vi "Main UI.vi"() -> ()   [LabVIEW 2021]
uses:
  subVIs/TypeDefs/UIControlReferences.ctl
  subVIs/TypeDefs/Tester Object.ctl
  <vilib>/NI/Modbus Library/API/Master/Modbus Master.lvclass
  <vilib>/Utility/error.llb/DialogType.ctl
panel:
  in  "Connect":bool
  in  "Stop Process":bool
  out "Equipment Status":bool caption="Equipment Connection"
  out "Positioning":dbl
  out "Motor Speed":dbl
  out "Temperature":dbl
  in  "ctrlCalibrate":bool
  out "Calibration":bool caption="Calibrated"
  in  "Sensibility Adjust":dbl caption="Sensibility"
  in  "ctrlSettingsButton":bool caption="Settings Button"
  in  "ctrlDirectionRotation":bool caption="Direction of Rotation"
  in  "ctrlMotorControlMode":bool caption="Motor Control Mode"
  in  "ctrlMotorControl":u16 caption="Motor Control (rpm)"
  in  "ctrlElevatorPosition":u16 caption="Elevator Position"
  in  "setShearRampStep":bool caption="Shear Ramp Step"
  in  "setOscillatory":bool caption="Oscillatory"
  in  "setShearRamp":bool caption="Shear Ramp"
  in  "setRTConstant":bool caption="Rotation or Torque Constant"
  in  "setElevatorPosition":bool caption="Set Elevator Position"
  in  "seqPauseButton":bool
  in  "Save Button":bool
  in  "stopJobSequence":bool
  in  "startJobSequence":bool
  in  "Data Analysis":bool
  in  "Job Sequence Tree":string(tree) caption="Job Sequence"
  out "XY Graph":cluster{dbl[], dbl[]}[](graph)
  out "Sensors":string[][](table)=[["Speed (rpm)", "125,6"], ["Torque (Nm)", "-0,301"], ["Height (mm)", "36"], ["Samples/s", "10,0"], ["Duration (s)", "250,4"]]
  out "Status String 3":string
  out "Status String 1":string
  out "Status String 2":string
  # "Equipment"
  # "Job Selection"
  # "Data Analysis"
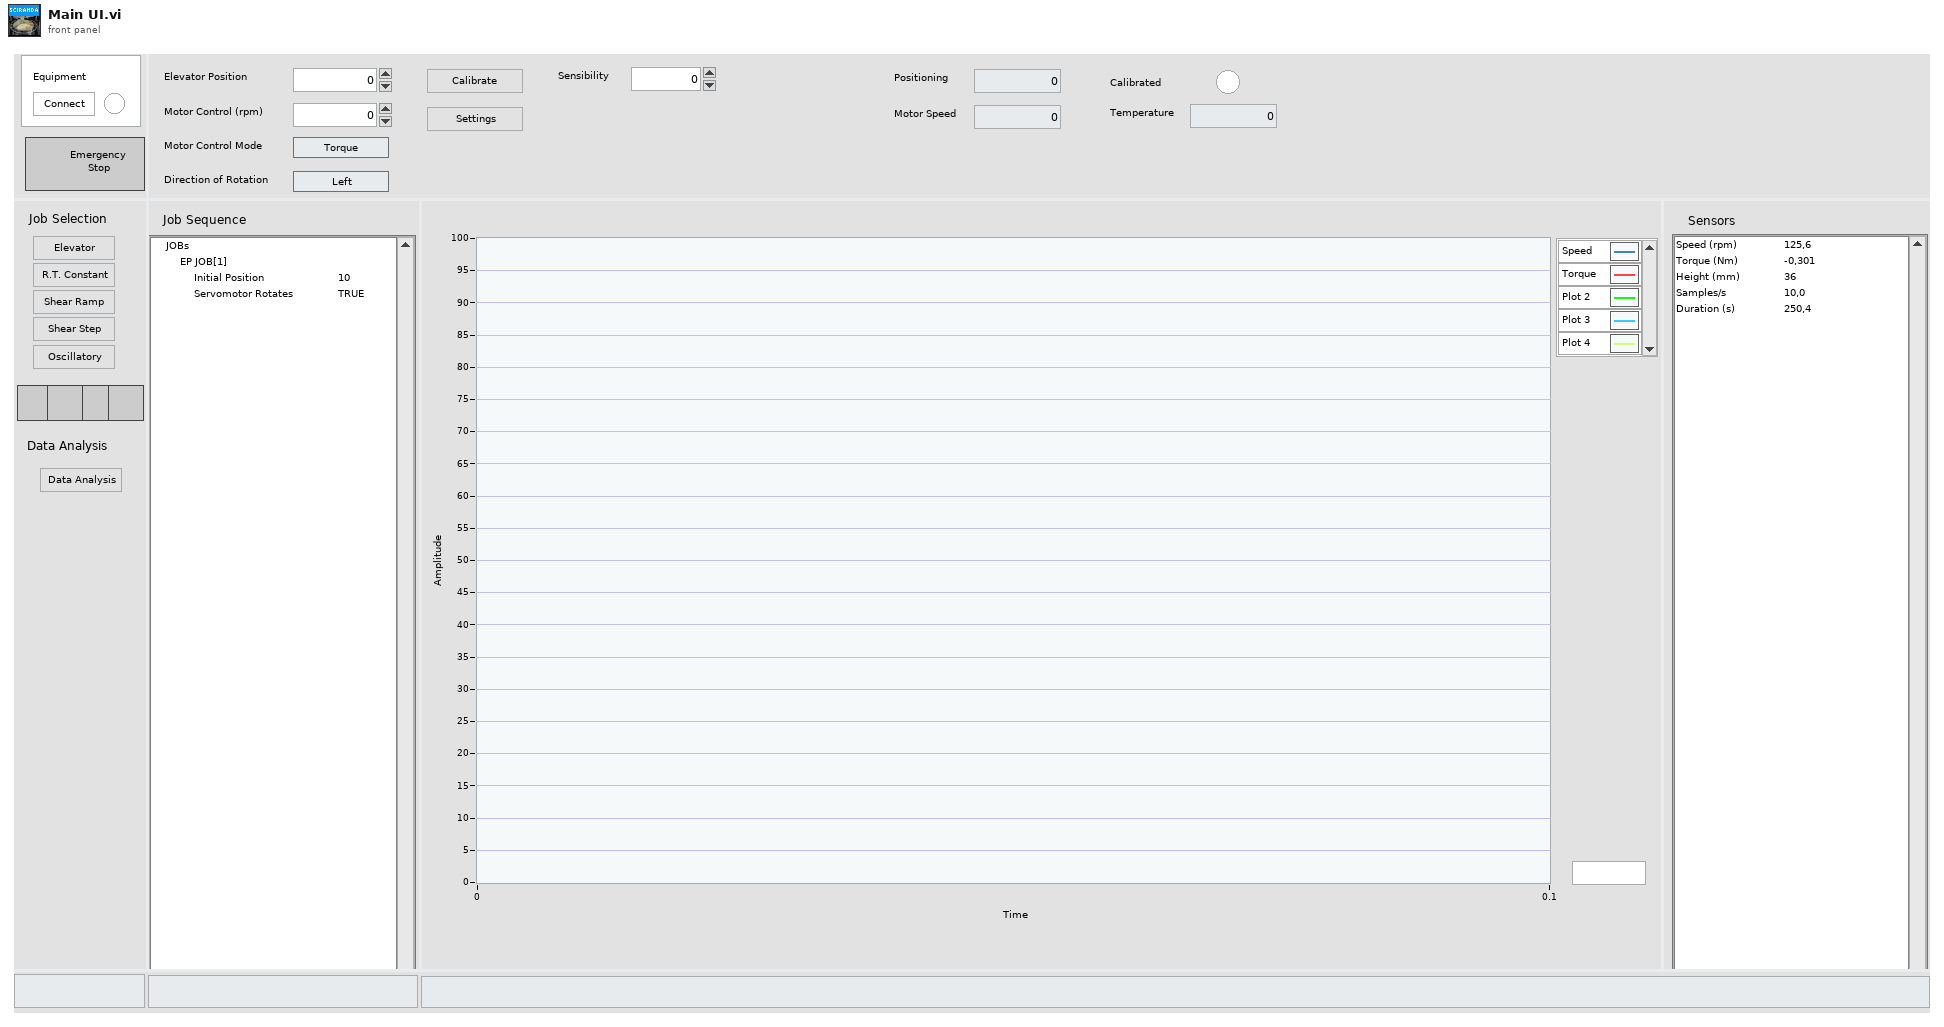
[diagram p1: front panel]
types:
  T1 = typedef "Tester Object.ctl" = cluster{"Program Properties":cluster{"Application Path":path}, "Control Refnum":T2, "Devices":cluster{"Modbus":cluster{"Modbus master instance":refnum<class "Modbus Master.lvclass">, "Modbus Address":cluster{"Session":string, cluster{"Key":string, "value":u32}[]}[]}, "TCP/IP":cluster{"connection ID":refnum<k5>, "Address":string}}}
  T2 = typedef "UIControlReferences.ctl" = cluster{"Tree Refnum ":refnum<vi>, "Graph1 Refnum":refnum<vi>, "Graph2 Refnum":refnum<vi>, "Temperature Refnum":refnum<vi>, "Sensor Str Refnum":refnum<vi>, "Motor Speed Refnum":refnum<vi>, "Equipment Connected Refnum":refnum<vi>, "Calibrated Refnum":refnum<vi>, "Positioning Refnum":refnum<vi>, "Servo On Refnum":refnum<vi>, "seqPauseButton":refnum<vi>, "seqStartButton":refnum<vi>, "seqStopButton":refnum<vi>}
  T3 = cluster{"Session":string, cluster{"Key":string, "value":u32}[]}[]
  T4 = typedef "DialogType.ctl" = u16
  T5 = cluster{"Modbus":cluster{"Modbus master instance":refnum<class "Modbus Master.lvclass">, "Modbus Address":cluster{"Session":string, cluster{"Key":string, "value":u32}[]}[]}, "TCP/IP":cluster{"connection ID":refnum<k5>, "Address":string}}
  T6 = typedef "ElevatorPositionConfiguration.ctl" = cluster{"ElevatorStartPosition":dbl, "ServomotorRotates":bool, "ElevatorPositionConfirmed?":bool}
  T7 = typedef "RotateOrTorqueConstantConfiguration.ctl" = cluster{"Constant Value":dbl, "Rotation or Torque":string, "Duration":dbl, "Confirmed?":bool}
  T8 = typedef "ShearRampConfiguration.ctl" = cluster{"Shear Ramp":string, "Rotation or Torque":string, "Initial Value":dbl, "Final Value":dbl, "Duration":dbl, "Number of Points":i32, "Confirmed?":bool, "Shear Ramp Array":dbl[][]}
  T9 = typedef "ShearRampStepConfiguration.ctl" = cluster{"Rotation or Torque":string, "Initial Value":dbl, "Final Value":dbl, "Step Duration":dbl, "Number of Steps":i32, "Shear Ramp Step Array":dbl[][], "Confirmed?":bool, "Shear Step Generation":enum16{"StepDurationConstant", "Table"}}
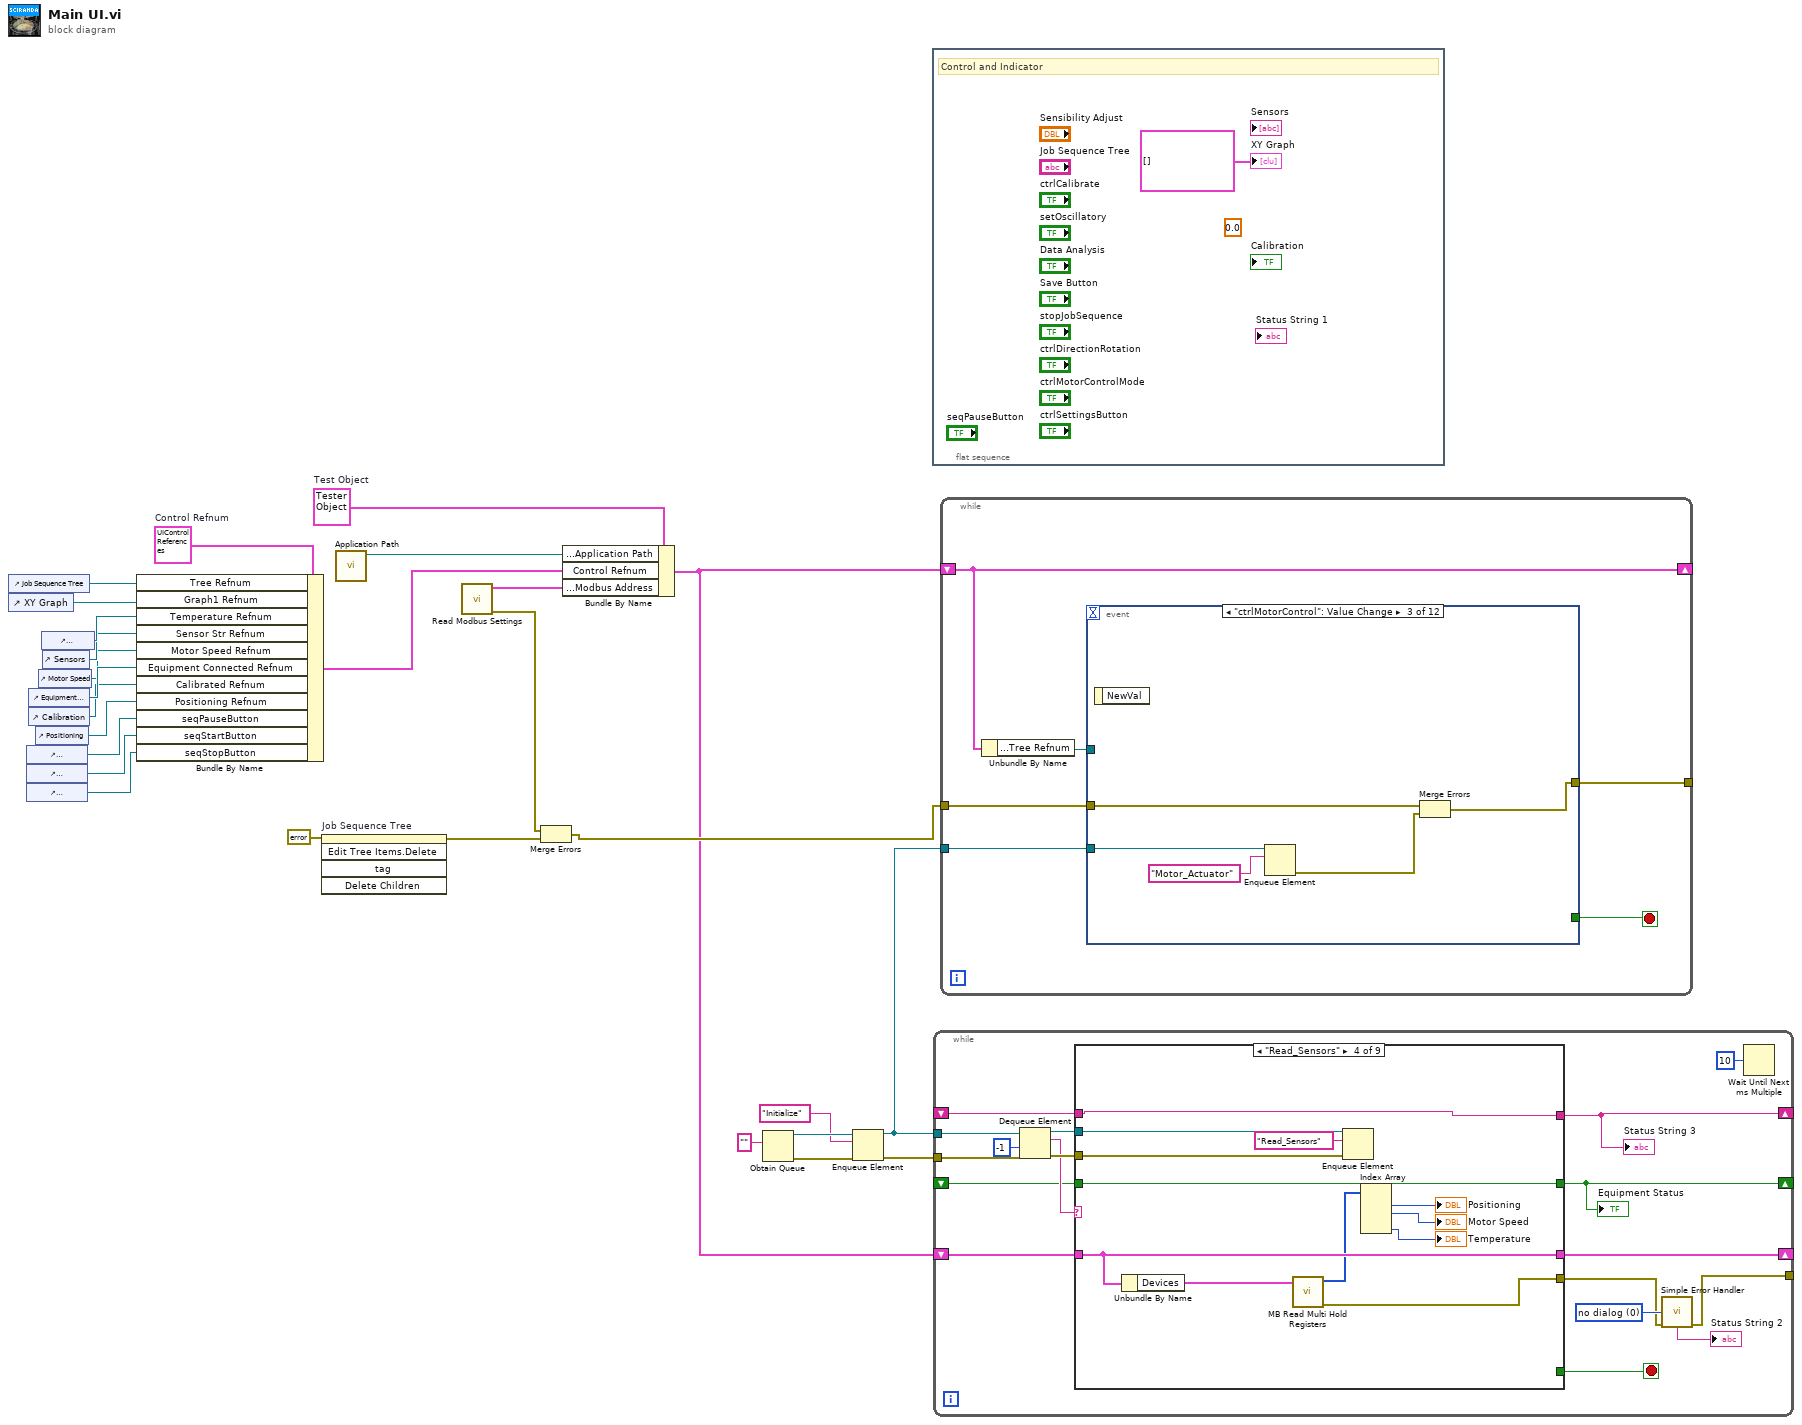
[diagram p0: block diagram]
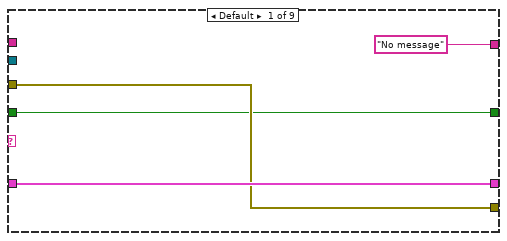
[diagram p2: hidden frame]
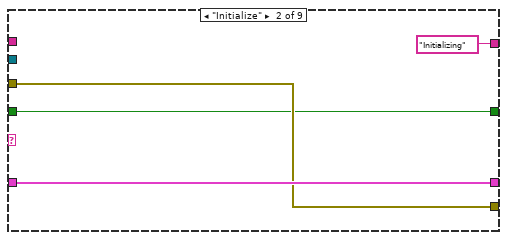
[diagram p3: hidden frame]
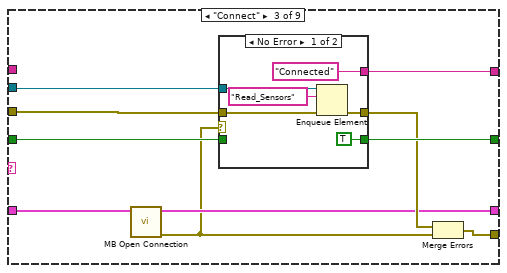
[diagram p4: hidden frame]
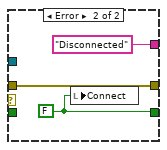
[diagram p5: hidden frame]
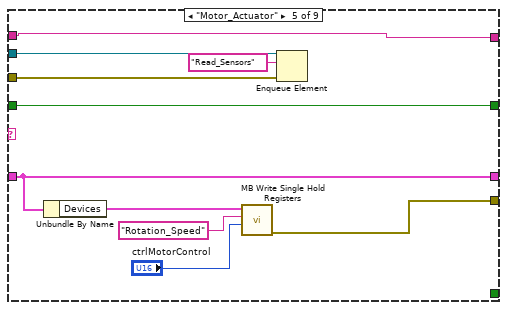
[diagram p6: hidden frame]
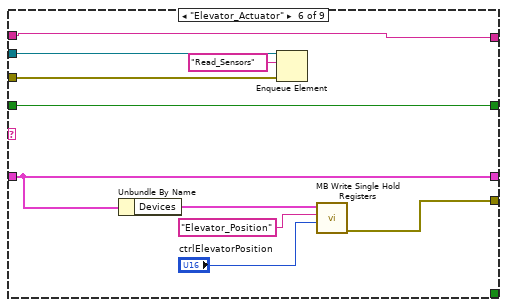
[diagram p7: hidden frame]
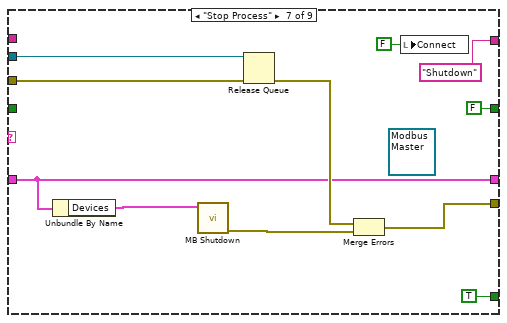
[diagram p8: hidden frame]
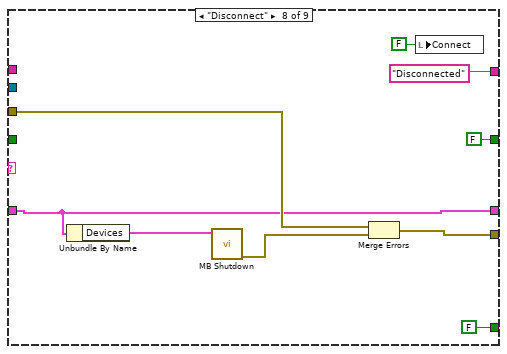
[diagram p9: hidden frame]
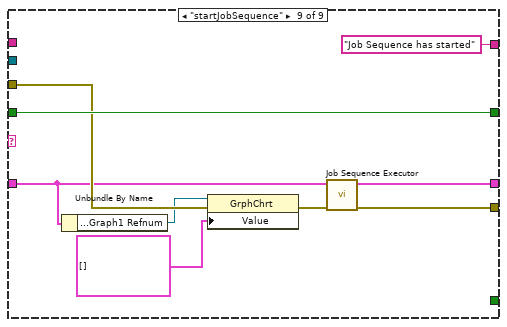
[diagram p10: hidden frame]
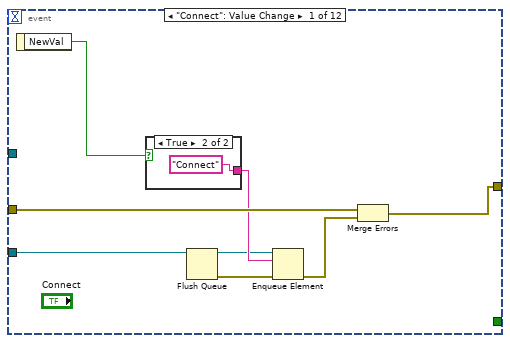
[diagram p11: hidden frame]
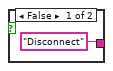
[diagram p12: hidden frame]
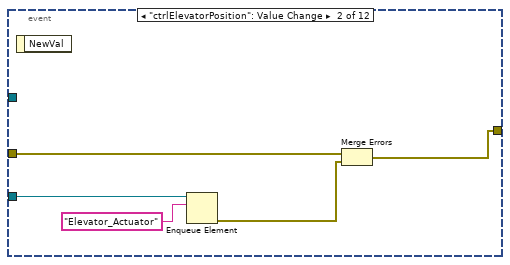
[diagram p13: hidden frame]
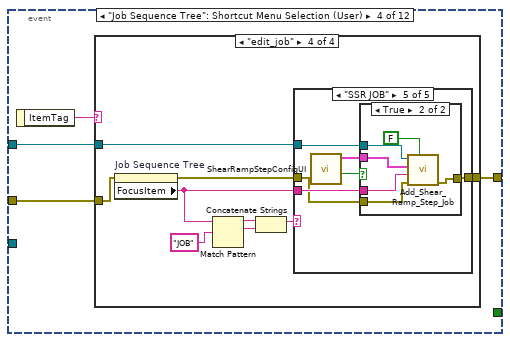
[diagram p14: hidden frame]
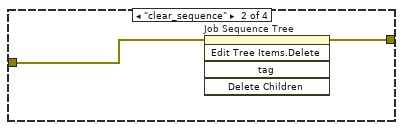
[diagram p16: hidden frame]
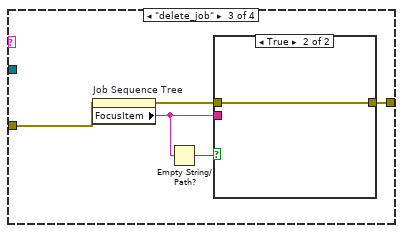
[diagram p17: hidden frame]
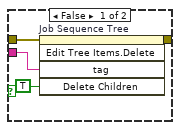
[diagram p18: hidden frame]
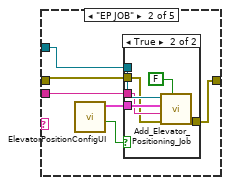
[diagram p20: hidden frame]
diagram:
  w10 = T1 {"Program Properties"={"Application Path"=path ""}, "Control Refnum"={"Tree Refnum "=refnum, "Graph1 Refnum"=refnum, "Graph2 Refnum"=refnum, "Temperature Refnum"=refnum, "Sensor Str Refnum"=refnum, "Motor Speed Refnum"=refnum, "Equipment Connected Refnum"=refnum, "Calibrated Refnum"=refnum, "Positioning Refnum"=refnum, "Servo On Refnum"=refnum, "seqPauseButton"=refnum, "seqStartButton"=refnum, "seqStopButton"=refnum}, "Devices"={"Modbus"={"Modbus master instance"=refnum, "Modbus Address"=[]}, "TCP/IP"={"connection ID"=refnum, "Address"=""}}}  # Test Object
  w20 = T2 {"Tree Refnum "=refnum, "Graph1 Refnum"=refnum, "Graph2 Refnum"=refnum, "Temperature Refnum"=refnum, "Sensor Str Refnum"=refnum, "Motor Speed Refnum"=refnum, "Equipment Connected Refnum"=refnum, "Calibrated Refnum"=refnum, "Positioning Refnum"=refnum, "Servo On Refnum"=refnum, "seqPauseButton"=refnum, "seqStartButton"=refnum, "seqStopButton"=refnum}  # Control Refnum
  n1 = control-ref of="Job Sequence Tree"() -> (w19:refnum<vi>)
  n2 = control-ref of="XY Graph"() -> (w14:refnum<vi>)
  n3 = control-ref of="seqPauseButton"() -> (w3:refnum<vi>)
  n4 = control-ref of="startJobSequence"() -> (w2:refnum<vi>)
  n5 = control-ref of="stopJobSequence"() -> (w1:refnum<vi>)
  n6 = control-ref of="Equipment Status"() -> (w16:refnum<vi>)
  n7 = control-ref of="Calibration"() -> (w15:refnum<vi>)
  n8 = control-ref of="Positioning"() -> (w5:refnum<vi>)
  n9 = control-ref of="Motor Speed"() -> (w4:refnum<vi>)
  n10 = control-ref of="Temperature"() -> (w18:refnum<vi>)
  n11 = control-ref of="Sensors"() -> (w17:refnum<vi>)
  n12 = Bundle By Name(cluster=w20, "Tree Refnum"=w19, "Graph1 Refnum"=w14, "Temperature Refnum"=w18, "Sensor Str Refnum"=w17, "Motor Speed Refnum"=w4, "Equipment Connected Refnum"=w16, "Calibrated Refnum"=w15, "Positioning Refnum"=w5, "seqPauseButton"=w3, "seqStartButton"=w2, "seqStopButton"=w1) -> (w9:T2)
  n13 = invoke on="Job Sequence Tree" class="Tree (strict)" method="Edit Tree Items.Delete"(error in=errorcluster {"status"=FALSE, "code"=0, "source"=""} ("error out")) -> (error out=w12:errorcluster)  [unwired: 4 in, 4 out]
  n14 = call "Application Path.vi"() -> ("appended path"=w7:path)  [unwired: 11 in]
  n15 = call "Read Modbus Settings.vi"() -> ("error out"=w11:errorcluster, "Ini File"=w6:T3)  [unwired: 10 in]
  n16 = Merge Errors(w11, w12) -> (w27:errorcluster)
  n17 = Bundle By Name(cluster=w10, "Program Properties.Application Path"=w7, "Control Refnum"=w9, "Devices.Modbus.Modbus Address"=w6) -> (w8:T1)
  n18 = Obtain Queue(element data type="" ("element")) -> (queue out=w26:refnum<queue>, error out=w24:errorcluster)  [unwired: 4 in, 1 out]
  n19 = Enqueue Element(queue=w26, element="Initialize", error in (no error)=w24) -> (queue out=w21:refnum<queue>, error out=w22:errorcluster)  [unwired: 1 in, 1 out]
  n20 = flat-sequence {
    frame #0 {
      (unwired) 0.0 ("Temperature")
      # "Control and Indicator"
      "XY Graph" <- cluster{dbl[], dbl[]}[] [] ("Multiplot XY Array")
    }
  }
  n21 = while {
    shift-right: [w45] -> _
    shift-left: w8 -> [w46]
    tunnel: w21 -> [w44]
    tunnel: w22 -> [w43]
    shift-right: [w38] -> _
    shift-left: _ -> [w37]
    tunnel: [w33] -> _
    shift-right: [w32] -> _
    shift-left: _ -> [w31]
    stop <- w39 stop-if-true
    w35 = T4 0 items=["no dialog", "OK message", "continue or stop message", "OK message + warnings", "continue/stop + warnings"] ("type of dialog (OK msg:1)")
    n22 = Dequeue Element(queue=w44, timeout in ms (-1)=-1, error in (no error)=w43) -> (queue out=w41:refnum<queue>, element=w40:string, error out=w42:errorcluster)  [unwired: 1 out]
    n23 = case shown="\"Read_Sensors\"" w40 {
      tunnel: w46 -> [w50 w54 w57 w80 w89 w98 w106 w117 w127]
      tunnel: [w48 w52 w63 w74 w95 w97 w115 w125 w132] -> w34
      tunnel: [w50 w54 w56 w80 w89 w98 w106 w117 w128] -> w45
      tunnel: w42 -> [w48 w52 w59 w82 w91 w102 w110 w120 w131]
      tunnel: w41 -> [_ _ w60 w83 w92 w103 w108 _ _]
      tunnel: ["No message" "Initializing" w64 w85 w94 w105 "Shutdown" "Disconnected" "Job Sequence has started"] -> w32
      tunnel: [_ _ _ _ _ _ TRUE FALSE _] -> w39
      tunnel: [w47 w51 w62 w84 w93 w104 FALSE FALSE w134] -> w38
      tunnel: w37 -> [w47 w51 w61 w84 w93 w104 _ _ w134]
      tunnel: w31 -> [_ _ _ w85 w94 w105 _ _ _]
      frame Default {
      }
      frame "Initialize" {
      }
      frame "Connect" {
        n24 = call "MB Open Connection.vi"("Test Object in"=w57) -> ("error out"=w55:errorcluster, "Test Object out"=w56:T1)  [unwired: 9 in]
        n25 = case shown="No Error" w55 {
          tunnel: ["Connected" "Disconnected"] -> w64
          tunnel: [TRUE w71] -> w62
          tunnel: w61 -> [_ _]
          tunnel: w60 -> [w68 _]
          tunnel: w59 -> [w67 w72]
          tunnel: [w65 w72] -> w58
          frame No Error {
            n26 = Enqueue Element(queue=w68, element="Read_Sensors", error in (no error)=w67) -> (error out=w65:errorcluster)  [unwired: 1 in, 2 out]
          }
          frame Error {
            w71 = FALSE
            n27 = local write "Connect"(w71) -> ()
          }
        }
        n28 = Merge Errors(w58, w55) -> (w63:errorcluster)
      }
      frame "Read_Sensors" {
        n29 = Unbundle By Name(w80) -> ("Devices"=w79:T5)
        n30 = call "MB Read Multi Hold Registers.vi"("Devices"=w79) -> ("error out"=w74:errorcluster, "Register Values"=w78:u16[])  [unwired: 9 in]
        n31 = Enqueue Element(queue=w83, element="Read_Sensors", error in (no error)=w82) -> ()  [unwired: 1 in, 3 out]
        n32 = Index Array(array=w78) -> (element #1=→"Positioning":u16, element #2=→"Motor Speed":u16, element #4=→"Temperature":u16)  [unwired: 4 in, 1 out]
      }
      frame "Motor_Actuator" {
        n33 = Unbundle By Name(w89) -> ("Devices"=w88:T5)
        n34 = call "MB Write Single Hold Registers.vi"("Write Hold Register"="ctrlMotorControl", "Control Variable"="Rotation_Speed", "Devices"=w88) -> ("error out"=w95:errorcluster)  [unwired: 7 in, 1 out]
        n35 = Enqueue Element(queue=w92, element="Read_Sensors", error in (no error)=w91) -> ()  [unwired: 1 in, 3 out]
      }
      frame "Elevator_Actuator" {
        n36 = Unbundle By Name(w98) -> ("Devices"=w100:T5)
        n37 = Enqueue Element(queue=w103, element="Read_Sensors", error in (no error)=w102) -> ()  [unwired: 1 in, 3 out]
        n38 = call "MB Write Single Hold Registers.vi"("Write Hold Register"="ctrlElevatorPosition", "Control Variable"="Elevator_Position", "Devices"=w100) -> ("error out"=w97:errorcluster)  [unwired: 7 in, 1 out]
      }
      frame "Stop Process" {
        (unwired) refnum<class "Modbus Master.lvclass"> refnum ("TCP master instance")
        n39 = Unbundle By Name(w106) -> ("Devices"=w107:T5)
        n40 = call "MB Shutdown.vi"("Devices"=w107) -> ("error out"=w116:errorcluster)  [unwired: 10 in]
        n41 = Release Queue(queue=w108, error in (no error)=w110) -> (error out=w109:errorcluster)  [unwired: 1 in, 2 out]
        n42 = Merge Errors(w109, w116) -> (w115:errorcluster)
        n43 = local write "Connect"(FALSE ("Connect")) -> ()
      }
      frame "Disconnect" {
        n44 = Unbundle By Name(w117) -> ("Devices"=w119:T5)
        n45 = call "MB Shutdown.vi"("Devices"=w119) -> ("error out"=w118:errorcluster)  [unwired: 10 in]
        n46 = Merge Errors(w120, w118) -> (w125:errorcluster)
        n47 = local write "Connect"(FALSE ("Connect")) -> ()
      }
      frame "startJobSequence" {
        n48 = Unbundle By Name(w127) -> ("Control Refnum.Graph1 Refnum"=w126:refnum<vi>)
        n49 = property class="GrphChrt"(reference=w126, error in=w131, "Value"=cluster{dbl[], dbl[]}[] [] ("Multiplot XY Array")) -> (error out=w130:errorcluster)  [unwired: 1 out]
        n50 = call "Job Sequence Executor.vi"("error out"=w130, "Test Object"=w127) -> ("error out 2"=w132:errorcluster, "Test Object out"=w128:T1)  [unwired: 8 in]
      }
    }
    "Equipment Status" <- w38
    "Status String 3" <- w32
    n51 = call <vilib>:"Simple Error Handler.vi"("type of dialog (OK msg:1)"=w35, "error in (no error)"=w34) -> ("error out"=w33:errorcluster, "message"=→"Status String 2":string)  [unwired: 3 in, 3 out]
    n52 = Wait Until Next ms Multiple(millisecond multiple=u32 10) -> ()  [unwired: 1 out]
  }
  n53 = while {
    tunnel: [w139] -> _
    tunnel: w27 -> [w138]
    tunnel: w21 -> [w137]
    shift-right: [w135] -> _
    shift-left: w8 -> [w135]
    stop <- w140 stop-if-true
    n54 = Unbundle By Name(w135) -> ("Control Refnum.Tree Refnum"=w136:refnum<vi>)
    n55 = event shown="[2] \"ctrlMotorControl\": Value Change" {
      selector: _ -> [_ _ _ _ _ _ _ _ _ _ _ _]
      dyn-events: _ -> [_ _ _ _ _ _ _ _ _ _ _ _]
      timeout: _ -> [_ _ _ _ _ _ _ _ _ _ _ _]
      tunnel: [_ _ _ _ FALSE FALSE FALSE FALSE _ TRUE _ TRUE] -> w140
      tunnel: [w146 w151 w156 w162 w243 w254 w265 w275 w286 w290 w297 w300] -> w139
      tunnel: w138 -> [w148 w153 w158 w163 w241 w253 w263 w274 w284 w291 w295 w301]
      tunnel: w137 -> [w143 w155 w160 _ _ _ _ _ w285 w293 _ w303]
      tunnel: w136 -> [_ _ _ w161 w240 w251 w262 w273 _ _ _ _]
      event "Connect": Value Change {
        n56 = event-data() -> ("NewVal"=w145:bool)  [unwired: 1 in]
        n57 = case shown="True" w145 {
          tunnel: ["Disconnect" ("element") "Connect" ("element")] -> w144
          frame False {
          }
          frame True {
          }
        }
        n58 = Flush Queue(queue=w143) -> (queue out=w142:refnum<queue>, error out=w141:errorcluster)  [unwired: 1 in, 1 out]
        n59 = Enqueue Element(queue=w142, element=w144, error in (no error)=w141) -> (error out=w147:errorcluster)  [unwired: 1 in, 2 out]
        n60 = Merge Errors(w148, w147) -> (w146:errorcluster)
      }
      event "ctrlElevatorPosition": Value Change {
        n61 = event-data() -> ()  [unwired: 1 in, 1 out]
        n62 = Enqueue Element(queue=w155, element="Elevator_Actuator") -> (error out=w152:errorcluster)  [unwired: 2 in, 2 out]
        n63 = Merge Errors(w153, w152) -> (w151:errorcluster)
      }
      event "ctrlMotorControl": Value Change {
        n64 = event-data() -> ()  [unwired: 1 in, 1 out]
        n65 = Enqueue Element(queue=w160, element="Motor_Actuator") -> (error out=w157:errorcluster)  [unwired: 2 in, 2 out]
        n66 = Merge Errors(w158, w157) -> (w156:errorcluster)
      }
      event "Job Sequence Tree": Shortcut Menu Selection (User) {
        n67 = event-data() -> ("ItemTag"=w164:string)  [unwired: 1 in]
        n68 = case shown="\"edit_job\"" w164 {
          tunnel: w163 -> [w165 w167 w171 w185]
          tunnel: [w165 w166 w172 w186] -> w162
          tunnel: w161 -> [_ _ _ w179]
          frame Default {
          }
          frame "clear_sequence" {
            n69 = invoke on="Job Sequence Tree" class="Tree (strict)" method="Edit Tree Items.Delete"(error in=w167) -> (error out=w166:errorcluster)  [unwired: 4 in, 4 out]
          }
          frame "delete_job" {
            n70 = property on="Job Sequence Tree" class="Tree (strict)"(error in=w171) -> (error out=w170:errorcluster, "FocusItem"=w169:string)  [unwired: 1 in, 1 out]
            n71 = Empty String/Path?(string/path=w169) -> (empty?=w168:bool)
            n72 = case shown="True" w168 {
              tunnel: [w176 w177] -> w172
              tunnel: w170 -> [w175 w177]
              tunnel: w169 -> [w173 _]
              frame False {
                n73 = invoke on="Job Sequence Tree" class="Tree (strict)" method="Edit Tree Items.Delete"(error in=w175, "tag"=w173, "Delete Children"=TRUE ("Delete Children?")) -> (error out=w176:errorcluster)  [unwired: 2 in, 4 out]
              }
              frame True {
              }
            }
          }
          frame "edit_job" {
            n74 = property on="Job Sequence Tree" class="Tree (strict)"(error in=w185) -> (error out=w184:errorcluster, "FocusItem"=w178:string)  [unwired: 1 in, 1 out]
            n75 = Match Pattern(string=w178, regular expression="JOB") -> (before substring=w181:string, match substring=w182:string)  [unwired: 1 in, 2 out]
            n76 = Concatenate Strings(w181, w182) -> (w180:string)
            n77 = case shown="\"SSR JOB\"" w180 {
              tunnel: [w187 w188 w204 w217 w228] -> w186
              tunnel: w184 -> [w187 w190 w201 w215 w229]
              tunnel: w179 -> [_ w193 w203 w216 w227]
              tunnel: w178 -> [_ w191 w202 w214 w230]
              frame Default {
              }
              frame "EP JOB" {
                n78 = call "ElevatorPositionConfigUI .vi"() -> ("Confirmed?"=w189:bool, "ElevatorPositionConfiguration"=w192:T6)  [unwired: 10 in]
                n79 = case shown="True" w189 {
                  tunnel: w193 -> [_ w200]
                  tunnel: w192 -> [_ w199]
                  tunnel: w191 -> [_ w197]
                  tunnel: w190 -> [w194 w196]
                  tunnel: [w194 w195] -> w188
                  frame False {
                  }
                  frame True {
                    n80 = call "Add_Elevator_Positioning_Job.vi"("New Job"=FALSE, "error in (no error)"=w196, "Item Edit"=w197, "ElevatorPositionConfiguration"=w199, "TreeControl in"=w200) -> ("error out"=w195:errorcluster)  [unwired: 5 in, 1 out]
                  }
                }
              }
              frame "RTC JOB" {
                n81 = call "RotationOrTorqueConstantConfigUI .vi"() -> ("Confirmed?"=w205:bool, "RotateOrTorqueConstantConfig"=w206:T7)  [unwired: 10 in]
                n82 = case shown="True" w205 {
                  tunnel: w206 -> [_ w213]
                  tunnel: [w207 w212] -> w204
                  tunnel: w203 -> [_ w210]
                  tunnel: w202 -> [_ w209]
                  tunnel: w201 -> [w207 w208]
                  frame False {
                  }
                  frame True {
                    n83 = call "Add_Constant_Speed_Movement_Job.vi"("New Job"=FALSE, "error in (no error)"=w208, "Tag Item"=w209, "RotateOrTorqueConstantConfig"=w213, "TreeControl in"=w210) -> ("error out"=w212:errorcluster)  [unwired: 5 in, 1 out]
                  }
                }
              }
              frame "LSR JOB" {
                n84 = call "ShearRampConfigUI .vi"() -> ("Confirmed?"=w218:bool, "ShearRampConfiguration"=w219:T8)  [unwired: 10 in]
                n85 = case shown="True" w218 {
                  tunnel: w219 -> [_ w226]
                  tunnel: w216 -> [_ w225]
                  tunnel: [w220 w224] -> w217
                  tunnel: w215 -> [w220 w223]
                  tunnel: w214 -> [_ w221]
                  frame False {
                  }
                  frame True {
                    n86 = call "Add_Shear_Ramp_Job.vi"("New Job"=FALSE, "error in (no error)"=w223, "Tag Item"=w221, "ShearRampConfiguration"=w226, "TreeControl in"=w225) -> ("error out"=w224:errorcluster)  [unwired: 6 in]
                  }
                }
              }
              frame "SSR JOB" {
                n87 = call "ShearRampStepConfigUI .vi"() -> ("Confirmed?"=w232:bool, "ShearRampConfiguration"=w231:T9)  [unwired: 10 in]
                n88 = case shown="True" w232 {
                  tunnel: w231 -> [_ w239]
                  tunnel: [w233 w238] -> w228
                  tunnel: w229 -> [w233 w237]
                  tunnel: w227 -> [_ w236]
                  tunnel: w230 -> [_ w235]
                  frame False {
                  }
                  frame True {
                    n89 = call "Add_Shear_Ramp_Step_Job.vi"("New Job"=FALSE, "error in (no error)"=w237, "Tag Item"=w235, "ShearRampStepConfiguration"=w239, "TreeControl in"=w236) -> ("error out"=w238:errorcluster)  [unwired: 6 in]
                  }
                }
              }
            }
          }
        }
      }
      event "setElevatorPosition": Value Change {
        n90 = event-data() -> ()  [unwired: 1 in, 1 out]
        n91 = call "ElevatorPositionConfigUI .vi"() -> ("Confirmed?"=w242:bool, "ElevatorPositionConfiguration"=w244:T6)  [unwired: 10 in]
        n92 = case shown="True" w242 {
          tunnel: w244 -> [_ w248]
          tunnel: w240 -> [_ w250]
          tunnel: [w246 w249] -> w243
          tunnel: w241 -> [w246 w247]
          frame False {
          }
          frame True {
            n93 = call "Add_Elevator_Positioning_Job.vi"("error in (no error)"=w247, "ElevatorPositionConfiguration"=w248, "TreeControl in"=w250) -> ("error out"=w249:errorcluster)  [unwired: 7 in, 1 out]
          }
        }
      }
      event "setRTConstant": Value Change {
        n94 = event-data() -> ()  [unwired: 1 in, 1 out]
        n95 = call "RotationOrTorqueConstantConfigUI .vi"() -> ("Confirmed?"=w252:bool, "RotateOrTorqueConstantConfig"=w255:T7)  [unwired: 10 in]
        n96 = case shown="True" w252 {
          tunnel: w255 -> [_ w261]
          tunnel: [w257 w260] -> w254
          tunnel: w251 -> [_ w259]
          tunnel: w253 -> [w257 w258]
          frame False {
          }
          frame True {
            n97 = call "Add_Constant_Speed_Movement_Job.vi"("error in (no error)"=w258, "RotateOrTorqueConstantConfig"=w261, "TreeControl in"=w259) -> ("error out"=w260:errorcluster)  [unwired: 7 in, 1 out]
          }
        }
      }
      event "setShearRamp": Value Change {
        n98 = event-data() -> ()  [unwired: 1 in, 1 out]
        n99 = call "ShearRampConfigUI .vi"() -> ("Confirmed?"=w264:bool, "ShearRampConfiguration"=w266:T8)  [unwired: 10 in]
        n100 = case shown="True" w264 {
          tunnel: w266 -> [_ w272]
          tunnel: w262 -> [_ w271]
          tunnel: [w268 w270] -> w265
          tunnel: w263 -> [w268 w269]
          frame False {
          }
          frame True {
            n101 = call "Add_Shear_Ramp_Job.vi"("error in (no error)"=w269, "ShearRampConfiguration"=w272, "TreeControl in"=w271) -> ("error out"=w270:errorcluster)  [unwired: 8 in]
          }
        }
      }
      event "setShearRampStep": Value Change {
        n102 = event-data() -> ()  [unwired: 1 in, 2 out]
        n103 = call "ShearRampStepConfigUI .vi"() -> ("Confirmed?"=w277:bool, "ShearRampConfiguration"=w276:T9)  [unwired: 10 in]
        n104 = case shown="True" w277 {
          tunnel: w276 -> [_ w283]
          tunnel: [w279 w282] -> w275
          tunnel: w274 -> [w279 w281]
          tunnel: w273 -> [_ w280]
          frame False {
          }
          frame True {
            n105 = call "Add_Shear_Ramp_Step_Job.vi"("error in (no error)"=w281, "ShearRampStepConfiguration"=w283, "TreeControl in"=w280) -> ("error out"=w282:errorcluster)  [unwired: 8 in]
          }
        }
      }
      event "startJobSequence": Value Change {
        n106 = event-data() -> ()  [unwired: 1 in, 1 out]
        n107 = Enqueue Element(queue=w285, element="startJobSequence") -> (error out=w287:errorcluster)  [unwired: 2 in, 2 out]
        n108 = Merge Errors(w284, w287) -> (w286:errorcluster)
      }
      event "Stop Process": Value Change {
        n109 = event-data() -> ()  [unwired: 1 in, 1 out]
        n110 = Enqueue Element At Opposite End(queue=w293, element="Stop Process") -> (error out=w292:errorcluster)  [unwired: 2 in, 2 out]
        n111 = Merge Errors(w291, w292) -> (w290:errorcluster)
      }
      event Menu Selection (User) {
        n112 = event-data() -> ("ItemTag"=w296:string)  [unwired: 1 in]
        n113 = case shown="\"modbus_settings_submenu\"" w296 {
          tunnel: [w298 w299] -> w297
          tunnel: w295 -> [w298 _]
          frame Default {
          }
          frame "modbus_settings_submenu" {
            n114 = call "Modbus UI Settings.vi"() -> ("error out"=w299:errorcluster)  [unwired: 11 in]
          }
        }
      }
      event Panel Close? {
        n115 = event-data() -> ()  [unwired: 1 in, 1 out]
        n116 = Enqueue Element At Opposite End(queue=w303, element="Stop Process", error in (no error)=w301) -> (error out=w300:errorcluster)  [unwired: 1 in, 2 out]
        n117 = event-data("Discard?"=TRUE) -> ()  [unwired: 1 in, 1 out]
      }
    }
  }
